vi "CANOpen PDO.vi"(8 "error in (no error)":errorcluster, 11 "Node Ptr":T1 format="%.0x") -> (0 "error out":errorcluster)   [LabVIEW 2021, in "CANOpen Addon System Explorer.lvlib"]
uses:
  CANOpen Addon System Explorer.lvlib
  <vilib>/NI VeriStand/Custom Device API/Custom Device Item Ref.ctl
  Shared/CANOpen Addon GUID Lookup Global.vi
  <vilib>/NI VeriStand/Custom Device API/Get Item Property (Variant).vi
  <vilib>/NI VeriStand/Custom Device API/Custom Device API.lvlib
  Shared/CANOpen Addon Shared.lvlib
panel:
  in  "PDO Channel":u8(ring)=1 items=["PDO 1", "PDO 2", "PDO 3", "PDO 4"]
  in  "SHDocVw.IWebBrowser2":refnum<k7>(container)
  in  "Header":cluster{"Section Name":string}={"Section Name"="PDOs"}
  in  "Description":string
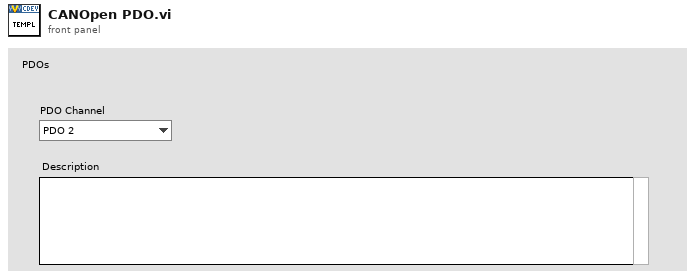
[diagram p1: front panel]
types:
  T1 = typedef "Custom Device API.lvlib/Custom Device Item Ref.ctl" = u64
  T2 = typedef "Custom Device API.lvlib/Custom Device Item Info.ctl" = cluster{"Name":string, "Is Channel":bool, "GUID":string, "Is Waveform":bool}
  T3 = typedef "Custom Device API.lvlib/Custom Device Commands.ctl" = enum16{"Default", "Item renamed", "Shutdown", "Dynamic button pressed"}
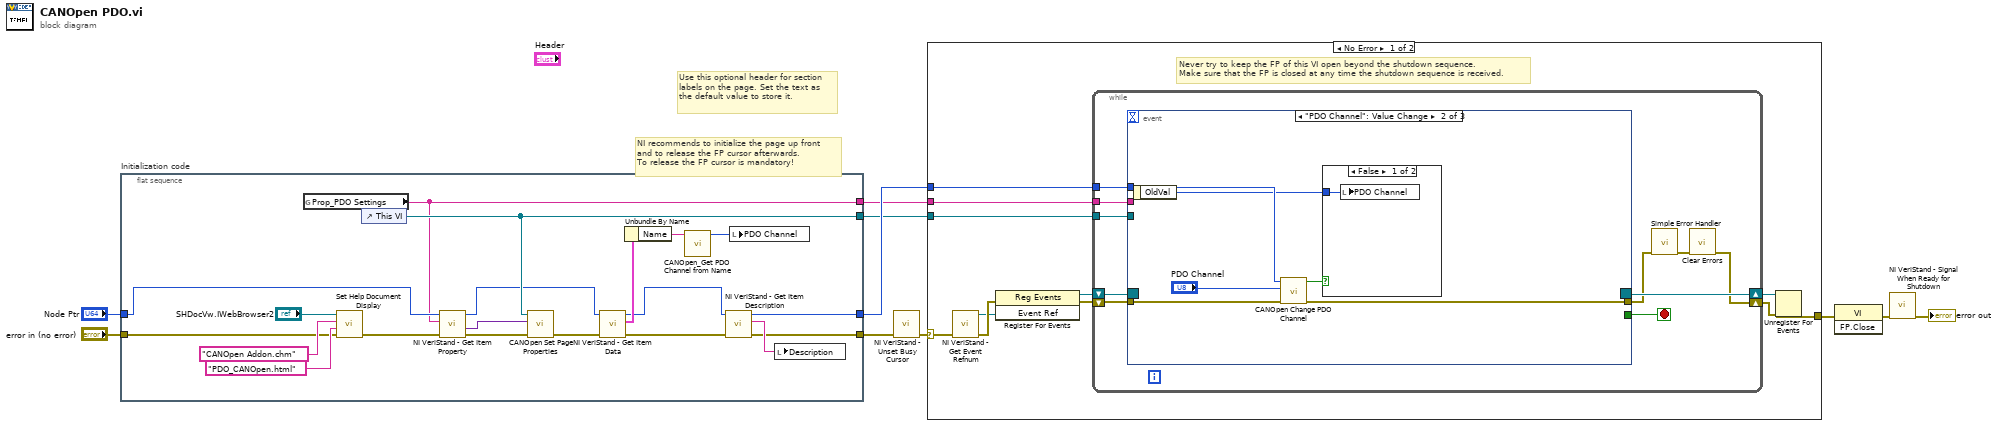
[diagram p0: block diagram]
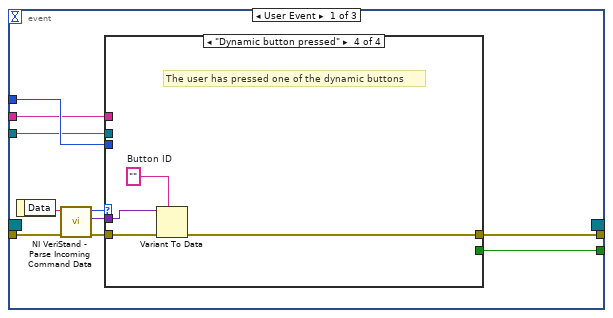
[diagram p2: hidden frame]
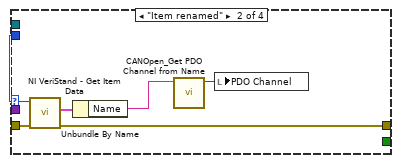
[diagram p4: hidden frame]
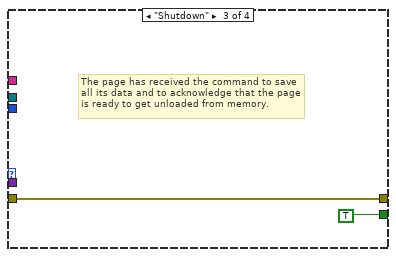
[diagram p5: hidden frame]
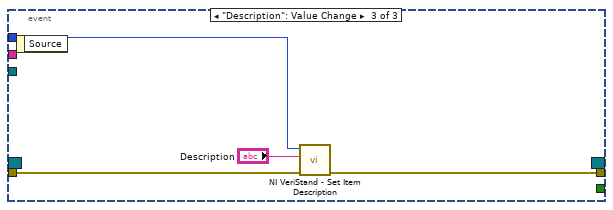
[diagram p7: hidden frame]
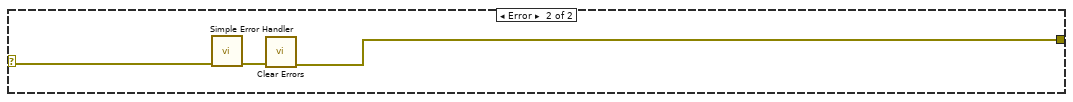
[diagram p8: hidden frame]
diagram:
  # "Use this optional header for section labels on the page. Set the text as the default value to store it."
  # "NI recommends to initialize the page up front\nand to release the FP cursor afterwards.\nTo release the FP cursor is mandatory!"
  n1 = flat-sequence "Initialization code" {
    tunnel: "error in (no error)" -> [w23]
    tunnel: "Node Ptr" -> [w22]
    tunnel: [w21] -> w6
    tunnel: [w20] -> w3
    tunnel: [w19] -> w2
    tunnel: [w18] -> w1
    frame #0 {
      n2 = global read "CANOpen Addon GUID Lookup Global.vi" "Prop_PDO Settings"() -> (w18:string)
      n3 = call "Set Help Document Display.vi"("error in (no error)"=w23, "HTML File"="PDO_CANOpen.html", "Main CHM File"="CANOpen Addon.chm", "SHDocVw.IWebBrowser2"="SHDocVw.IWebBrowser2") -> ("error out"=w27:errorcluster)  [unwired: 7 in]
      n4 = control-ref of="This VI"() -> (w19:refnum<vi>)
      n5 = call-poly <vilib>:"NI VeriStand - Get Item Property.vi"("error in (no error)"=w27, "Property Name"=w18, "Item Ref in"=w22) -> ("error out"=w29:errorcluster, "Value"=w28:variant, "Item Ref out"=w14:T1)  [unwired: 5 in, 1 out]
      n6 = call "CANOpen Set Page Properties.vi"("error in"=w29, "variant"=w28, "This VI"=w19) -> ("error out"=w16:errorcluster)  [unwired: 8 in]
      n7 = call <vilib>:"NI VeriStand - Get Item Data.vi"("error in (no error)"=w16, "Item Ref in"=w14) -> ("error out"=w15:errorcluster, "Item Info"=w17:T2, "Item Ref out"=w13:T1)  [unwired: 7 out]
      n8 = Unbundle By Name(w17) -> ("Name"=w12:string)
      n9 = call "CANOpen_Get PDO Channel from Name.vi"("PDO Channel Name"=w12) -> ("PDO Channel"=w11:i32)  [unwired: 10 in]
      n10 = call <vilib>:"NI VeriStand - Get Item Description.vi"("error in (no error)"=w15, "Item Ref in"=w13) -> ("error out"=w21:errorcluster, "Description"=w30:string, "Item Ref out"=w20:T1)  [unwired: 7 out]
      n11 = local write "PDO Channel"(w11) -> ()
      n12 = local write "Description"(w30) -> ()
    }
  }
  n13 = call <vilib>:"NI VeriStand - Unset Busy Cursor.vi"("error in (no error)"=w6) -> ("error out"=w5:errorcluster)  [unwired: 10 out]
  n14 = case shown="No Error" w5 {
    selector: w5 -> [w33 w88]
    tunnel: [w38 w86] -> w10
    tunnel: w3 -> [w34 _]
    tunnel: w2 -> [w32 _]
    tunnel: w1 -> [w31 _]
    frame No Error {
      # "Never try to keep the FP of this VI open beyond the shutdown sequence.\nMake sure that the FP is closed at any time the shutdown sequence is received."
      n15 = call <vilib>:"NI VeriStand - Get Event Refnum.vi"("error in (no error)"=w33) -> ("error out"=w41:errorcluster, "Event Ref"=w37:refnum<user-event>)  [unwired: 9 out]
      n16 = register-events(error in=w41, w37) -> (reference out=w35:refnum<event-registration>, error out=w36:errorcluster)  [unwired: 1 in]
      n17 = while {
        tunnel: w34 -> [w47]
        shift-right: [w44] -> w39
        shift-left: w36 -> [w50]
        shift-right: [w51] -> w40
        shift-left: w35 -> [w49]
        tunnel: w32 -> [w43]
        tunnel: w31 -> [w42]
        stop <- w48 stop-if-true
        n18 = event shown="[1] \"PDO Channel\": Value Change" {
          selector: w49 -> [_ _ _]
          dyn-events: [_ _ _] -> w51
          timeout: _ -> [_ _ _]
          tunnel: w50 -> [w61 w80 w84]
          tunnel: [w57 _ _] -> w48
          tunnel: [w56 w78 w83] -> w46
          tunnel: w47 -> [w55 w77 w85]
          tunnel: w43 -> [w53 _ _]
          tunnel: w42 -> [w52 _ _]
          event User Event {
            n19 = event-data() -> ("Data"=w60:string)  [unwired: 1 out]
            n20 = call <vilib>:"NI VeriStand - Parse Incoming Command Data.vi"("error in (no error)"=w61, "Incoming data"=w60) -> ("error out"=w59:errorcluster, "Outgoing data"=w54:variant, "Action"=w58:T3)  [unwired: 7 out]
            n21 = case shown="\"Dynamic button pressed\"" w58 {
              tunnel: w59 -> [w62 w68 w69 w74]
              tunnel: [_ _ TRUE _] -> w57
              tunnel: [w62 w65 w69 w71] -> w56
              tunnel: w55 -> [_ w67 _ _]
              tunnel: w54 -> [_ _ _ w73]
              tunnel: w53 -> [_ _ _ _]
              tunnel: w52 -> [_ _ _ _]
              frame "Default", Default {
              }
              frame "Item renamed" {
                n22 = call <vilib>:"NI VeriStand - Get Item Data.vi"("error in (no error)"=w68, "Item Ref in"=w67) -> ("error out"=w65:errorcluster, "Item Info"=w66:T2)  [unwired: 8 out]
                n23 = Unbundle By Name(w66) -> ("Name"=w64:string)
                n24 = call "CANOpen_Get PDO Channel from Name.vi"("PDO Channel Name"=w64) -> ("PDO Channel"=w63:i32)  [unwired: 10 in]
                n25 = local write "PDO Channel"(w63) -> ()
              }
              frame "Shutdown" {
                # "The page has received the command to save all its data and to acknowledge that the page is ready to get unloaded from memory."
              }
              frame "Dynamic button pressed" {
                w72 = ""  # Button ID
                # "The user has pressed one of the dynamic buttons"
                n26 = Variant To Data(error in=w74, type=w72, Variant=w73) -> (error out=w71:errorcluster)  [unwired: 1 out]
              }
            }
          }
          event "PDO Channel": Value Change {
            n27 = event-data() -> ("OldVal"=w75:u8)  [unwired: 1 out]
            n28 = call "CANOpen Change PDO Channel.vi"("error in (no error)"=w80, "PDO Channel"="PDO Channel", "Node Ptr"=w77) -> ("error out"=w78:errorcluster, "Passed?"=w76:bool)  [unwired: 7 in]
            n29 = case shown="False" w76 {
              tunnel: w75 -> [w81 _]
              frame False {
                n30 = local write "PDO Channel"(w81) -> ()
              }
              frame True {
              }
            }
          }
          event "Description": Value Change {
            n31 = event-data() -> ()  [unwired: 2 out]
            n32 = call <vilib>:"NI VeriStand - Set Item Description.vi"("error in (no error)"=w84, "Description"="Description", "Item Ref in"=w85) -> ("error out"=w83:errorcluster)  [unwired: 8 out]
          }
        }
        n33 = call <vilib>:"Simple Error Handler.vi"("error in (no error)"=w46) -> ("error out"=w45:errorcluster)  [unwired: 1 in, 7 out]
        n34 = call <vilib>:"Clear Errors.vi"("error in (no error)"=w45) -> ("error out"=w44:errorcluster)  [unwired: 1 in, 5 out]
      }
      n35 = Unregister For Events(event registration refnum=w40, error in=w39) -> (error out=w38:errorcluster)
    }
    frame Error {
      n36 = call <vilib>:"Simple Error Handler.vi"("error in (no error)"=w88) -> ("error out"=w87:errorcluster)  [unwired: 1 in, 7 out]
      n37 = call <vilib>:"Clear Errors.vi"("error in (no error)"=w87) -> ("error out"=w86:errorcluster)  [unwired: 1 in, 5 out]
    }
  }
  n38 = invoke class="VI" method="FP.Close"(error in=w10) -> (error out=w9:errorcluster)  [unwired: 2 in, 2 out]
  n39 = call <vilib>:"NI VeriStand - Signal When Ready for Shutdown.vi"("error in (no error)"=w9) -> ("error out"=→"error out":errorcluster)  [unwired: 10 out]
